vi "LcString_XmlEnumToStringValue.vi"(0 "XmlEnumStringIn":string, 1 "EnumVariantIn(used if String is Empty)":variant, 5 "error in (no error)":errorcluster) -> (14 "EnumValueOut(string)":string, 15 "EnumItems(string)":string[](array[string]), 16 "EnumValueOut(uint16)":u16, 19 "error out":errorcluster)   [LabVIEW 2019]
doc: "Uses a flatten XML string of a Enum-type <B>\"XmlEnumStringIn\"</B> to find the acctually value of the enum.\nThis is normally used when a Enum has been flatten to a variant.\nIt could also take the enum variant as an input\nIt the Variant ENUM is of string type it will send it through without any errors"
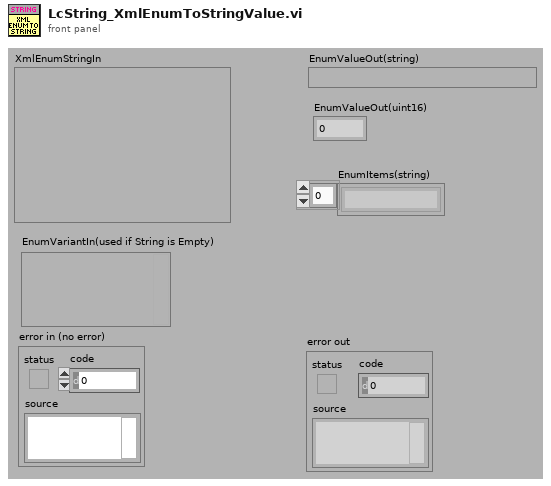
[diagram p1: front panel]
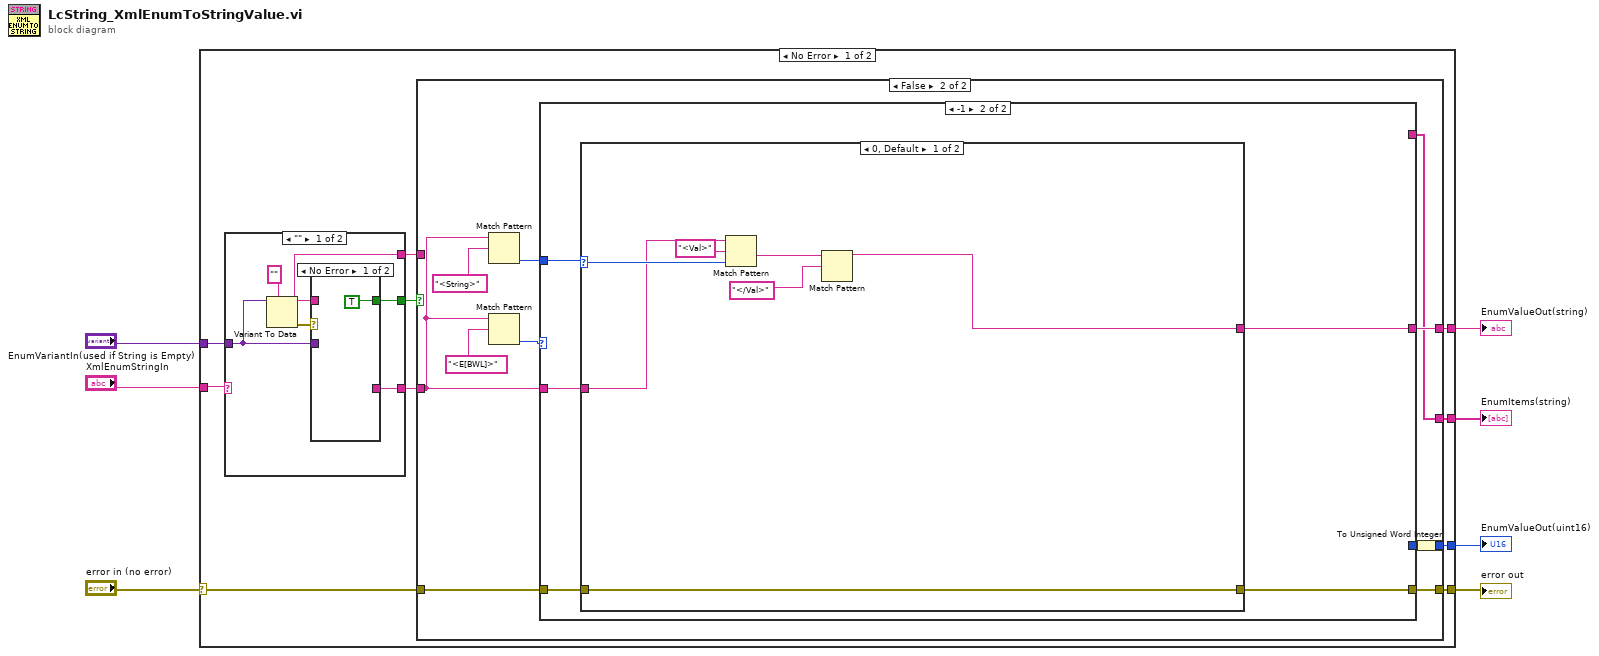
[diagram p0: block diagram]
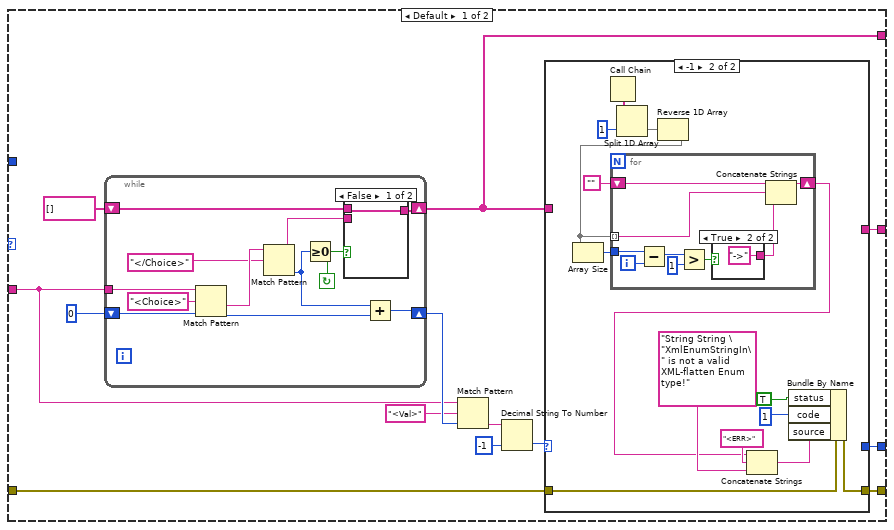
[diagram p3: hidden frame]
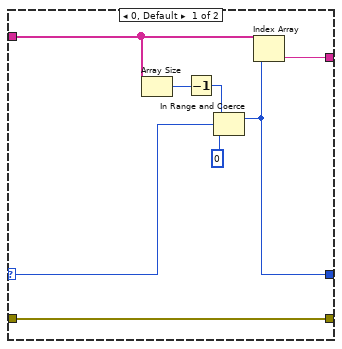
[diagram p4: hidden frame]
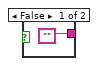
[diagram p5: hidden frame]
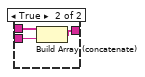
[diagram p6: hidden frame]
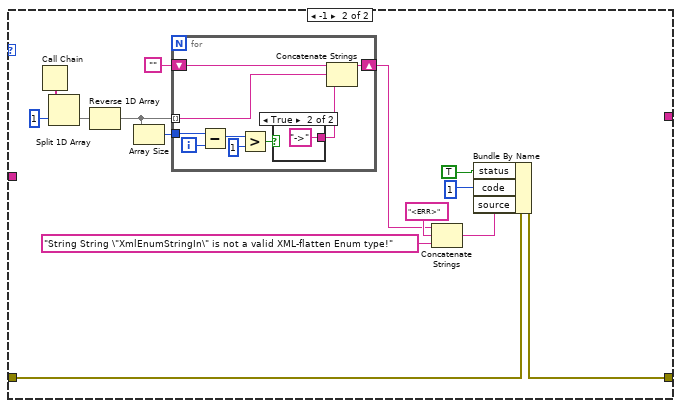
[diagram p7: hidden frame]
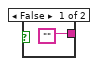
[diagram p8: hidden frame]
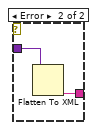
[diagram p9: hidden frame]
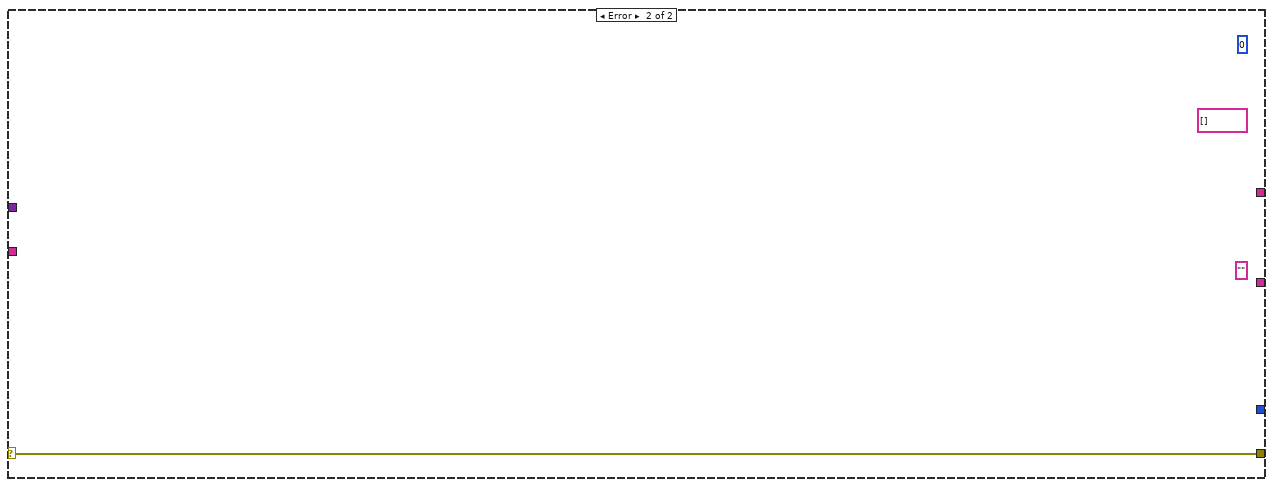
[diagram p11: hidden frame]
diagram:
  n1 = case shown="No Error" "error in (no error)" {
    selector: "error in (no error)" -> [w17 w140]
    tunnel: [w16 w140] -> w6
    tunnel: "XmlEnumStringIn" -> [w13 _]
    tunnel: [w15 _] -> w4
    tunnel: [w14 _] -> w3
    tunnel: "EnumVariantIn(used if String is Empty)" -> [w12 _]
    tunnel: [w10 _] -> w1
    frame No Error {
      n2 = case shown="\"\"" w13 {
        selector: w13 -> [_ w139]
        tunnel: [w135 w139] -> w11
        tunnel: w12 -> [w134 _]
        tunnel: [w131 _] -> w9
        tunnel: [w130 _] -> w8
        frame "" {
          n3 = Variant To Data(type="", Variant=w134) -> (data=w131:string, error out=w132:errorcluster)  [unwired: 1 in]
          n4 = case shown="No Error" w132 {
            tunnel: [_ w138] -> w135
            tunnel: w134 -> [_ w137]
            tunnel: w131 -> [_ _]
            tunnel: [TRUE _] -> w130
            frame No Error {
            }
            frame Error {
              n5 = Flatten To XML(anything=w137) -> (xml string=w138:string)
            }
          }
        }
        frame Default {
        }
      }
      n6 = case shown="False" w8 {
        tunnel: w17 -> [w18 w28]
        tunnel: [w18 w27] -> w16
        tunnel: [w19 w26] -> w15
        tunnel: [_ w24] -> w14
        tunnel: w11 -> [_ w22]
        tunnel: [_ w20] -> w10
        tunnel: w9 -> [w19 _]
        frame True {
        }
        frame False {
          n7 = Match Pattern(string=w22, regular expression="<String>") -> (offset past match=w21:i32)  [unwired: 4 out]
          n8 = Match Pattern(string=w22, regular expression="<E[BWL]>") -> (offset past match=w29:i32)  [unwired: 4 out]
          n9 = case shown="-1" w29 {
            tunnel: w22 -> [w40 w93]
            tunnel: w28 -> [w35 w97]
            tunnel: [w34 w96] -> w27
            tunnel: [w33 w94] -> w26
            tunnel: [w32 _] -> w25
            tunnel: w21 -> [_ w95]
            tunnel: [w31 _] -> w20
            frame Default {
              n10 = while {
                shift-left: 0 ("offset past match") -> [w86]
                shift-right: [w82] -> w41
                tunnel: w40 -> [w87]
                shift-right: [w78] -> w31
                shift-left: string[] [] -> [w79]
                stop <- w80 continue-if-true
                n11 = Match Pattern(string=w87, regular expression="<Choice>", offset (0)=w86) -> (after substring=w85:string, offset past match=w83:i32)  [unwired: 2 out]
                n12 = Match Pattern(string=w85, regular expression="</Choice>") -> (before substring=w77:string, offset past match=w81:i32)  [unwired: 3 out]
                n13 = Greater Or Equal To 0?(x=w81) -> (x >= 0?=w80:bool)
                n14 = case shown="False" w80 {
                  tunnel: w79 -> [w89 w92]
                  tunnel: [w89 w91] -> w78
                  tunnel: w77 -> [_ w90]
                  frame False {
                  }
                  frame True {
                    n15 = Build Array (concatenate)(w92, w90) -> (w91:string[])
                  }
                }
                n16 = Add(x=w81, y=w83) -> (x+y=w82:i32)
              }
              n17 = Match Pattern(string=w40, regular expression="<Val>", offset (0)=w41) -> (after substring=w38:string)  [unwired: 3 out]
              n18 = Decimal String To Number(string=w38, default (0L)=-1 ("default (0 I32)")) -> (number=w36:i32)  [unwired: 2 out]
              n19 = case shown="-1" w36 {
                selector: w36 -> [w46 _]
                tunnel: w35 -> [w51 w62]
                tunnel: [w51 w59] -> w34
                tunnel: w31 -> [w49 _]
                tunnel: [w50 _] -> w33
                tunnel: [w45 _] -> w32
                frame 0, Default {
                  n20 = Array Size(array=w49) -> (size(s)=w48:i32)
                  n21 = Decrement(x=w48) -> (x-1=w47:i32)
                  n22 = In Range and Coerce(upper limit=w47, x=w46, lower limit=0) -> (coerced(x)=w45:i32)  [unwired: 1 out]
                  n23 = Index Array(array=w49, index=w45) -> (element=w50:string)
                }
                frame -1 {
                  n24 = Call Chain() -> (call chain=w58:string[])
                  n25 = Split 1D Array(array=w58, index=1) -> (second subarray=w56:string[])  [unwired: 1 out]
                  n26 = Reverse 1D Array(array=w56) -> (reversed array=w53:string[])
                  n27 = Array Size(array=w53) -> (size(s)=w55:i32)
                  n28 = for {
                    shift-right: [w66] -> w52
                    shift-left: "" -> [w69]
                    tunnel: w53 -> [w67] mode=indexing
                    tunnel: w55 -> [w74]
                    i -> [w73]
                    n29 = Subtract(x=w74, y=w73) -> (x-y=w72:i32)
                    n30 = Greater?(x=w72, y=1) -> (0:w70:bool)
                    n31 = case shown="True" w70 {
                      tunnel: ["" "->"] -> w68
                      frame False {
                      }
                      frame True {
                      }
                    }
                    n32 = Concatenate Strings(w69, w67, w68) -> (w66:string)
                  }
                  n33 = Concatenate Strings(w52, "<ERR>" ("Substring"), "String String \"XmlEnumStringIn\" is not a valid XML-flatten Enum type!" ("source")) -> (w64:string)
                  n34 = Bundle By Name(cluster=w62, "status"=TRUE ("Bundle Element"), "code"=1 ("code (5000)"), "source"=w64) -> (w59:errorcluster)
                }
              }
            }
            frame -1 {
              n35 = case shown="0, Default" w95 {
                selector: w95 -> [w103 _]
                tunnel: w97 -> [w99 w113]
                tunnel: [w99 w114] -> w96
                tunnel: [w100 _] -> w94
                tunnel: w93 -> [w98 _]
                frame 0, Default {
                  n36 = Match Pattern(string=w98, regular expression="<Val>", offset (0)=w103) -> (after substring=w102:string)  [unwired: 3 out]
                  n37 = Match Pattern(string=w102, regular expression="</Val>") -> (before substring=w100:string)  [unwired: 4 out]
                }
                frame -1 {
                  n38 = Call Chain() -> (call chain=w111:string[])
                  n39 = Split 1D Array(array=w111, index=1) -> (second subarray=w109:string[])  [unwired: 1 out]
                  n40 = Reverse 1D Array(array=w109) -> (reversed array=w106:string[])
                  n41 = Array Size(array=w106) -> (size(s)=w108:i32)
                  n42 = for {
                    shift-right: [w119] -> w105
                    shift-left: "" -> [w122]
                    tunnel: w106 -> [w120] mode=indexing
                    tunnel: w108 -> [w127]
                    i -> [w126]
                    n43 = Subtract(x=w127, y=w126) -> (x-y=w125:i32)
                    n44 = Greater?(x=w125, y=1) -> (0:w123:bool)
                    n45 = case shown="True" w123 {
                      tunnel: ["" "->"] -> w121
                      frame False {
                      }
                      frame True {
                      }
                    }
                    n46 = Concatenate Strings(w122, w120, w121) -> (w119:string)
                  }
                  n47 = Concatenate Strings(w105, "<ERR>" ("Substring"), "String String \"XmlEnumStringIn\" is not a valid XML-flatten Enum type!" ("source")) -> (w117:string)
                  n48 = Bundle By Name(cluster=w113, "status"=TRUE ("Bundle Element"), "code"=1 ("code (5000)"), "source"=w117) -> (w114:errorcluster)
                }
              }
            }
          }
          n49 = To Unsigned Word Integer(number=w25) -> (unsigned 16bit integer=w24:u16)
        }
      }
    }
    frame Error {
      (unwired) string[] []
      (unwired) 0
      (unwired) "" ("String in")
    }
  }
  "error out" <- w6
  "EnumValueOut(string)" <- w4
  "EnumValueOut(uint16)" <- w3
  "EnumItems(string)" <- w1
